vi "Launch Freezer Actor.vi"(0 "Caller Actor in":refnum<class "Actor.lvclass">, 1 "Thresholds":cluster{"Upper":dbl, "Lower":dbl}={"Upper"=0.1, "Lower"=-0.8}, 2 "Name":string="Freezer", 3 "DedicatedEnQrs":refnum<queue>, 5 "SHVs":T2, 9 "Heater":T1=enum."Undefined", 11 "error in (no error)":errorcluster, 12 "Interlock Chain":refnum<class "Interlock Chain.lvclass">, 14 "Low Temp (-170)":dbl=-170.0 format="%#_13g") -> (4 "Caller-To-Actor Enqueuer":refnum<class "Message Enqueuer.lvclass">, 15 "error out":errorcluster)   [LabVIEW 2015, in "cRIO-Carbondioxide.lvlib" / "CO2-Actor.lvlib" / "Freezer.lvclass"]
uses:
  Actors/Freezer/Freezer.lvclass
  <vilib>/ActorFramework/Message Enqueuer/Message Enqueuer.lvclass
  <vilib>/ActorFramework/Actor/Actor.lvclass
  Interlocks/Interlock Chain/Interlock Chain.lvclass
  Actors/cRIO-CO2/Blowers Heaters Enumerator.ctl
  Controls/Dedicated Enqueuers.ctl
  Actors/CO2 Actor/CO2 Actor.lvclass
  Actors/Freezer/Freezer.lvclass/Freezer.ctl
  Actors/cRIO-CO2/cRIO-CO2.lvclass
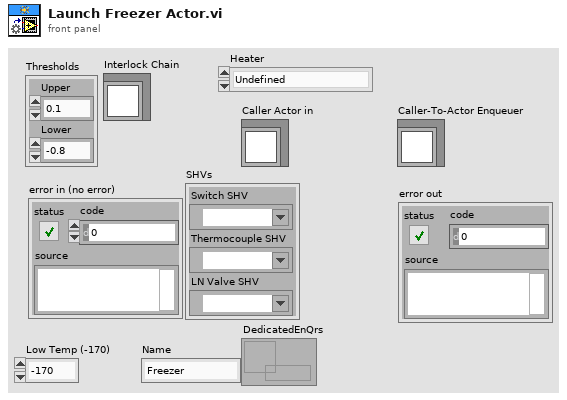
[diagram p1: front panel]
types:
  T1 = typedef "cRIO-Carbondioxide.lvlib/cRIO-CO2.lvlib/cRIO-CO2.lvclass/Blowers Heaters Enumerator.ctl" = enum16{"Tank Blower 1", "Tank Blower 2", "Tank Blower 3", "Tank Blower 4", "Syringe Blower", "Syringe Heater", "Piston Heater", "Undefined"}
  T2 = cluster{"Switch SHV":refnum<k21>, "Thermocouple SHV":refnum<k21>, "LN Valve SHV":refnum<k21>}
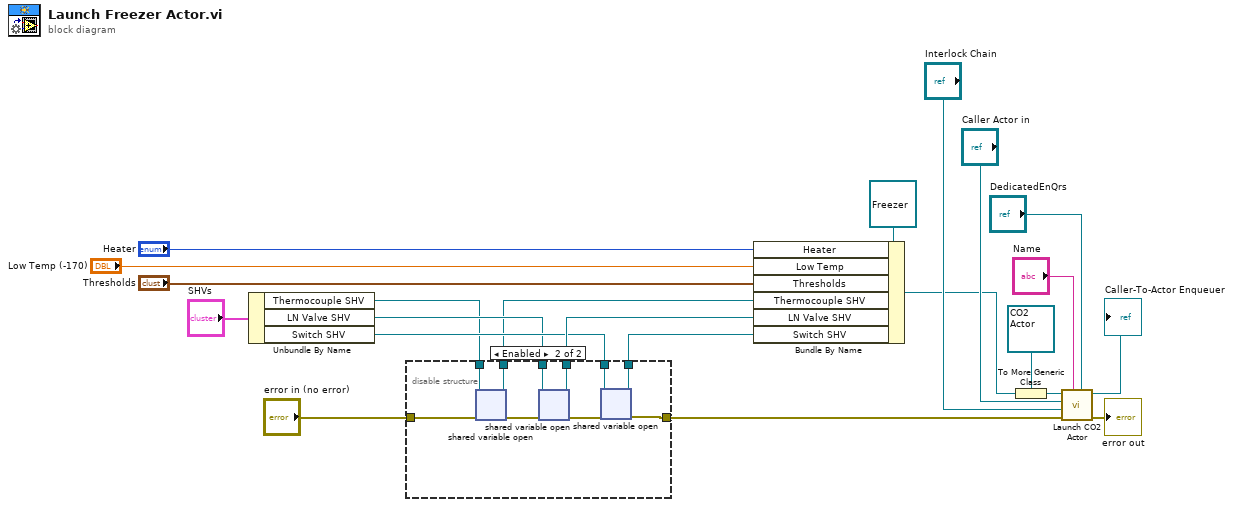
[diagram p0: block diagram]
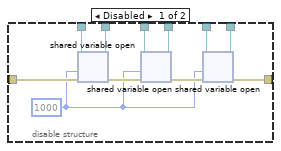
[diagram p2: hidden frame]
diagram:
  n1 = Unbundle By Name("SHVs") -> ("Thermocouple SHV"=w12:refnum<k21>, "LN Valve SHV"=w13:refnum<k21>, "Switch SHV"=w14:refnum<k21>)
  n2 = disable-structure shown="Enabled" {
    disable-tunnel: "error in (no error)" -> [w33 w43]
    disable-tunnel: [w31 w36] -> w19
    disable-tunnel: [w29 w34] -> w16
    disable-tunnel: w14 -> [w27 w35]
    disable-tunnel: w13 -> [w26 w37]
    disable-tunnel: w12 -> [w25 w42]
    disable-tunnel: [w24 w41] -> w11
    disable-tunnel: [w23 w38] -> w9
    frame Disabled {
      w28 = 1000 ("timeout ms")
      n3 = shared-variable-open(w25, w33, w28) -> (w24:refnum<k21>, w32:errorcluster)  [unwired: 2 in]
      n4 = shared-variable-open(w26, w32, w28) -> (w31:refnum<k21>, w30:errorcluster)  [unwired: 2 in]
      n5 = shared-variable-open(w27, w30, w28) -> (w29:refnum<k21>, w23:errorcluster)  [unwired: 1 in]
    }
    frame Enabled {
      n6 = shared-variable-open(w42, w43) -> (w41:refnum<k21>, w40:errorcluster)  [unwired: 1 in]
      n7 = shared-variable-open(w37, w40) -> (w36:refnum<k21>, w39:errorcluster)  [unwired: 1 in]
      n8 = shared-variable-open(w35, w39) -> (w34:refnum<k21>, w38:errorcluster)
    }
  }
  n9 = Bundle By Name(cluster=refnum<class "Freezer.lvclass"> refnum ("Freezer.lvclass"), "Heater"="Heater", "Low Temp"="Low Temp (-170)", "Thresholds"="Thresholds", "Thermocouple SHV"=w11, "LN Valve SHV"=w19, "Switch SHV"=w16) -> (w4:refnum<class "Freezer.lvclass">)
  n10 = To More Generic Class(target class=refnum<class "CO2 Actor.lvclass"> refnum ("CO2 Actor in"), reference=w4) -> (generic class reference=w5:refnum<class "CO2 Actor.lvclass">)
  n11 = call "Launch CO2 Actor.vi"("DedicatedEnQrs"="DedicatedEnQrs", "Name"="Name", "error in (no error)"=w9, "Interlock Chain"="Interlock Chain", "Caller Actor in"="Caller Actor in", "CO2 Actor in"=w5) -> ("error out"=→"error out":errorcluster, "Caller-To-Actor Enqueuer"=→"Caller-To-Actor Enqueuer":refnum<class "Message Enqueuer.lvclass">)  [unwired: 4 in]
